vi "retrieveStateData.vi"(7 "Target? (F)":bool, 8 "error in (no error)":errorcluster, 11 "statemachine in":refnum<class "statemachine.lvclass">) -> (0 "error out":errorcluster, 1 "State Data":refnum<class "data.lvclass">, 2 "State":refnum<class "state.lvclass">, 3 "statemachine out":refnum<class "statemachine.lvclass">)   [LabVIEW 2020, in "eos.lvlib" / "statemachine.lvclass"]
uses:
  statemachine.lvclass
  interfaces/state/state.lvclass
  interfaces/data/data.lvclass
  statemachine.lvclass/statemachine.ctl
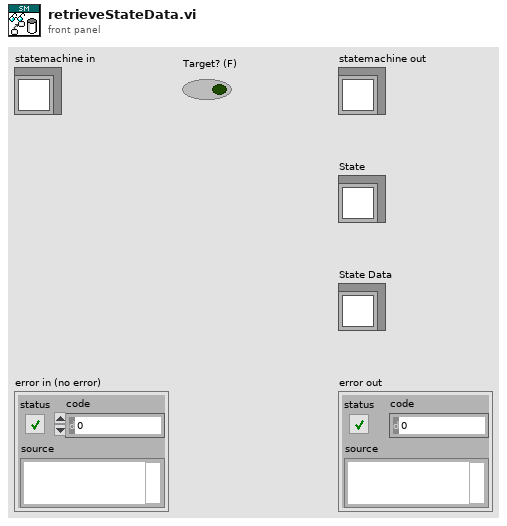
[diagram p1: front panel]
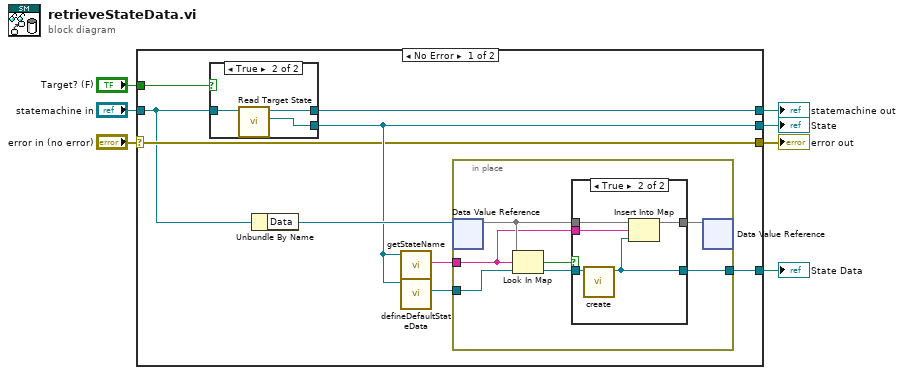
[diagram p0: block diagram]
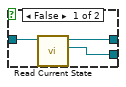
[diagram p2: hidden frame]
diagram:
  n1 = case shown="No Error" "error in (no error)" {
    selector: "error in (no error)" -> [w12 w37]
    tunnel: [w8 _] -> w2
    tunnel: "statemachine in" -> [w10 w38]
    tunnel: [w11 w38] -> w4
    tunnel: [w13 _] -> w6
    tunnel: [w12 w37] -> w7
    tunnel: "Target? (F)" -> [w9 _]
    frame No Error {
      n2 = case shown="True" w9 {
        tunnel: [w19 w20] -> w13
        tunnel: [w18 w21] -> w11
        tunnel: w10 -> [w17 w22]
        frame False {
          n3 = call "Read Current State.vi"("statemachine in"=w17) -> ("Current State"=w19:refnum<class "state.lvclass">, "statemachine out"=w18:refnum<class "statemachine.lvclass">)  [unwired: 9 in]
        }
        frame True {
          n4 = call "Read Target State.vi"("statemachine in"=w22) -> ("Target State"=w20:refnum<class "state.lvclass">, "statemachine out"=w21:refnum<class "statemachine.lvclass">)  [unwired: 9 in]
        }
      }
      n5 = Unbundle By Name(w10) -> ("Data"=w16:refnum<data-value>)
      n6 = call-dynamic "getStateName.vi"("state in"=w13) -> ("State Name"=w14:string)  [unwired: 8 in, 2 out]
      n7 = call-dynamic "defineDefaultStateData.vi"("state in"=w13) -> ("Default State Data"=w15:refnum<class "data.lvclass">)  [unwired: 8 in, 2 out]
      n8 = in-place {
        in-place-border: w14 -> [w23]
        in-place-border: w15 -> [w29]
        in-place-border: [w24] -> w8
        n9 = in-place-dvr #1(w16) -> (w28:map{string, refnum<class "data.lvclass">})  [unwired: 1 out]
        n10 = Look In Map(map=w28, key=w23, default value=w29) -> (key not found?=w27:bool, value=w26:refnum<class "data.lvclass">)
        n11 = case shown="True" w27 {
          tunnel: w26 -> [w31 w36]
          tunnel: [w31 w33] -> w24
          tunnel: w28 -> [w30 w35]
          tunnel: [w30 w32] -> w25
          tunnel: w23 -> [_ w34]
          frame False {
          }
          frame True {
            n12 = call-dynamic "create.vi"("data in"=w36) -> ("data out"=w33:refnum<class "data.lvclass">)  [unwired: 9 in, 1 out]
            n13 = Insert Into Map(map in=w35, key=w34, value=w33) -> (map out=w32:map{string, refnum<class "data.lvclass">})  [unwired: 2 out]
          }
        }
        n14 = in-place-dvr #1(w25) -> ()  [unwired: 2 out]
      }
    }
    frame Error {
    }
  }
  "error out" <- w7
  "State" <- w6
  "statemachine out" <- w4
  "State Data" <- w2
